vi "G_mobileye_Temp.vi"() -> ()   [LabVIEW 2015]
panel:
  out "lane_left 2":dbl[][](array[numeric])
  out "lane_right 2":dbl[][](array[numeric])
  out "lane_right":dbl[](array[numeric])
  out "lane_left":dbl[](array[numeric])
  out "obs":dbl[][](array[numeric])
  out "mobileye time":u32
  out "y_m_r":dbl[](array[numeric])
  out "y_m_l":dbl[](array[numeric])
  out "x_m":dbl[](array[numeric])
  out "y_obs":dbl[](array[numeric])
  out "x_obs":dbl[](array[numeric])
  out "y_l":dbl[](array[numeric])
  out "x_l":dbl[](array[numeric])
  out "y_r":dbl[](array[numeric])
  out "x_r":dbl[](array[numeric])
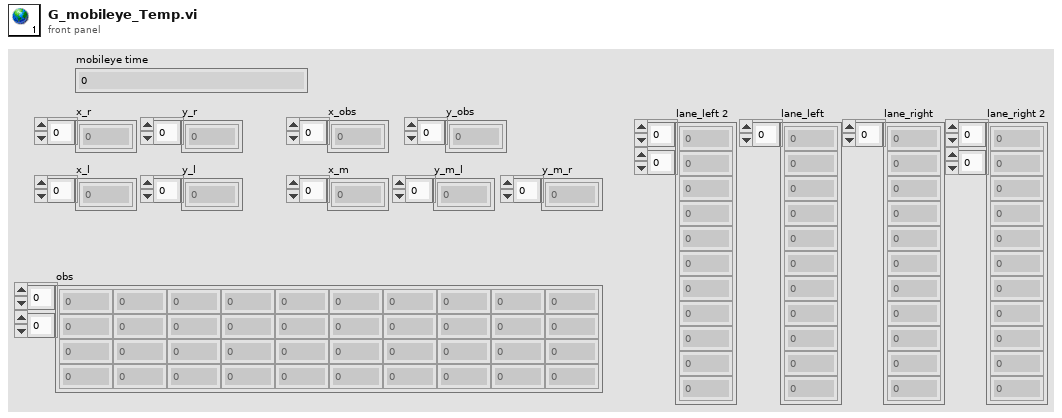
[diagram p1: front panel]
diagram:
